vi "Get Position.vi"(8 "error in (no error)":errorcluster, 10 "Axis":i32=1, 11 "ESP301 in":refnum<class "ESP301.lvclass">) -> (0 "error out":errorcluster, 1 "Position":dbl, 3 "ESP301 out":refnum<class "ESP301.lvclass">)   [LabVIEW 2019, in "ESP301.lvclass"]
uses:
  ESP301.lvclass
  ESP301.lvclass/ESP301.ctl
  ESP301-Driver/ESP301-Driver.lvlib
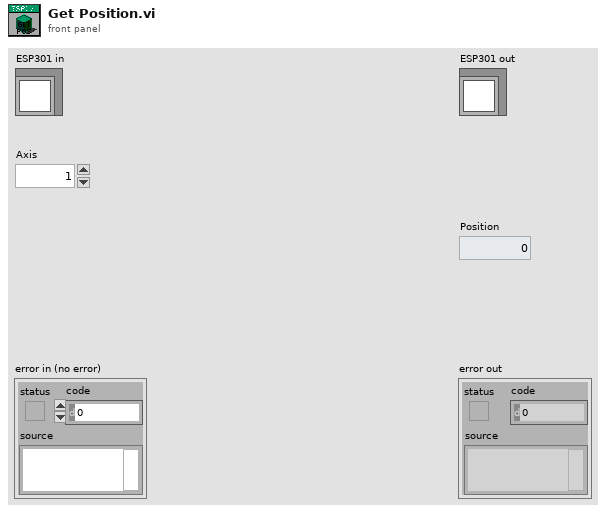
[diagram p1: front panel]
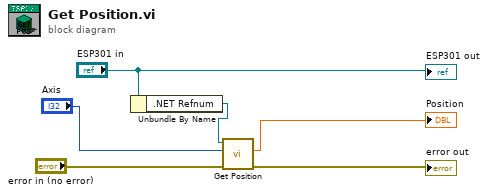
[diagram p0: block diagram]
diagram:
  n1 = Unbundle By Name("ESP301 in") -> (".NET Refnum"=w2:refnum<k24>)
  n2 = call "Get Position.vi"("error in (no error)"="error in (no error)", "Axis"="Axis", ".NET Refnum in"=w2) -> ("error out"=→"error out":errorcluster, "position"=→"Position":dbl)  [unwired: 6 in, 1 out]
  "ESP301 out" <- "ESP301 in"
